vi "Check if Error or Channel Controls.vi"(11 "Label.Text":string) -> (2 "Error?":bool, 3 "offset past match":i32)   [LabVIEW 2021, in "Converter.lvlib"]
uses:
  Converter.lvlib
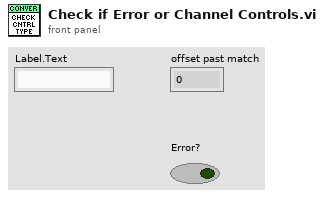
[diagram p1: front panel]
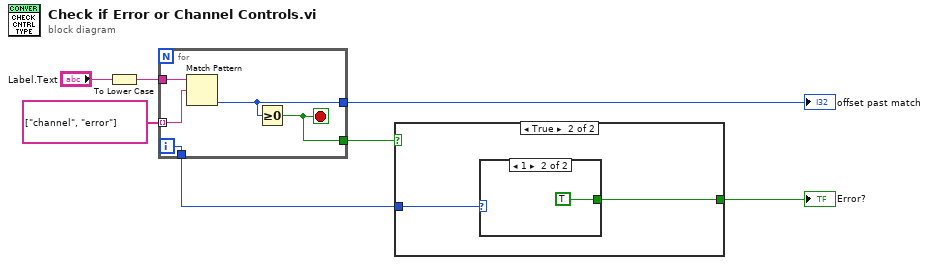
[diagram p0: block diagram]
diagram:
  n1 = To Lower Case(string="Label.Text") -> (all lower case string=w6:string)
  n2 = for {
    tunnel: w6 -> [w12]
    tunnel: [w10] -> w4
    tunnel: string[] ["channel", "error"] ("regular expression") -> [w11] mode=indexing
    tunnel: [w9] -> w3
    tunnel: [w8] -> w2
    i -> [w8]
    stop <- w9 stop-if-true
    n3 = Match Pattern(string=w12, regular expression=w11) -> (offset past match=w10:i32)  [unwired: 1 in, 3 out]
    n4 = Greater Or Equal To 0?(x=w10) -> (x >= 0?=w9:bool)
  }
  "offset past match" <- w4
  n5 = case shown="True" w3 {
    tunnel: w2 -> [_ w14]
    tunnel: [_ w13] -> w1
    frame False {
    }
    frame True {
      n6 = case shown="1" w14 {
        tunnel: [_ TRUE] -> w13
        frame Default {
        }
        frame 1 {
        }
      }
    }
  }
  "Error?" <- w1
